vi "IQramp.vi"(8 "Q counter":fxp<+/-,14,14> format="%#_8f", 9 "I counter":fxp<+/-,13,13> format="%#_8f", 10 "cos":fxp<+/-,16,0>, 11 "sin":fxp<+/-,16,0>) -> (0 "Q counter out":fxp<+/-,14,14>, 1 "I counter out":fxp<+/-,13,13>, 3 "signal":i16)   [LabVIEW 2013]
uses:
  <vilib>/rvi/FXPMathLib/FxpConvert/subVIs/nifxpmath_Convert_SimConfig.ctl
  <vilib>/fxp/LVFixedPointQuantizationPolicyTypeDef.ctl
  <vilib>/fxp/LVFixedPointOverflowPolicyTypeDef.ctl
  <vilib>/rvi/FXPMathLib/FxpConvert/simVIs/DllFxpConvertTemp_sub.vi
  <vilib>/rvi/FXPMathLib/FxpInterpret/XNode/nifxpmath_Interpret.xnode
  <vilib>/rvi/FXPMathLib/FxpConvert/XNode/nifxpmath_Convert.xnode
  <vilib>/rvi/FXPMathLib/FxpMul/XNode/nifxpmath_Multiplier.xnode
  <vilib>/rvi/FXPMathLib/FxpSub/XNode/nifxpmath_Sub.xnode
  <vilib>/rvi/FXPMathLib/FxpAdd/XNode/nifxpmath_Add.xnode
  <vilib>/rvi/FXPMathLib/sim/FxpSim.dll
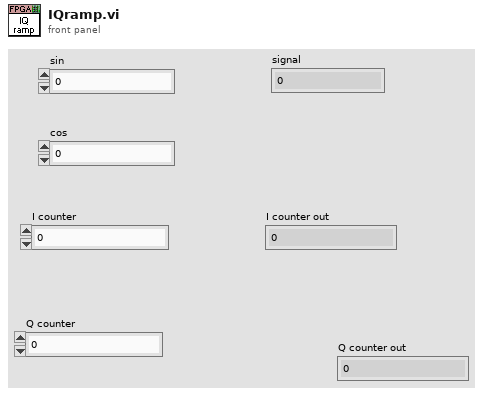
[diagram p1: front panel]
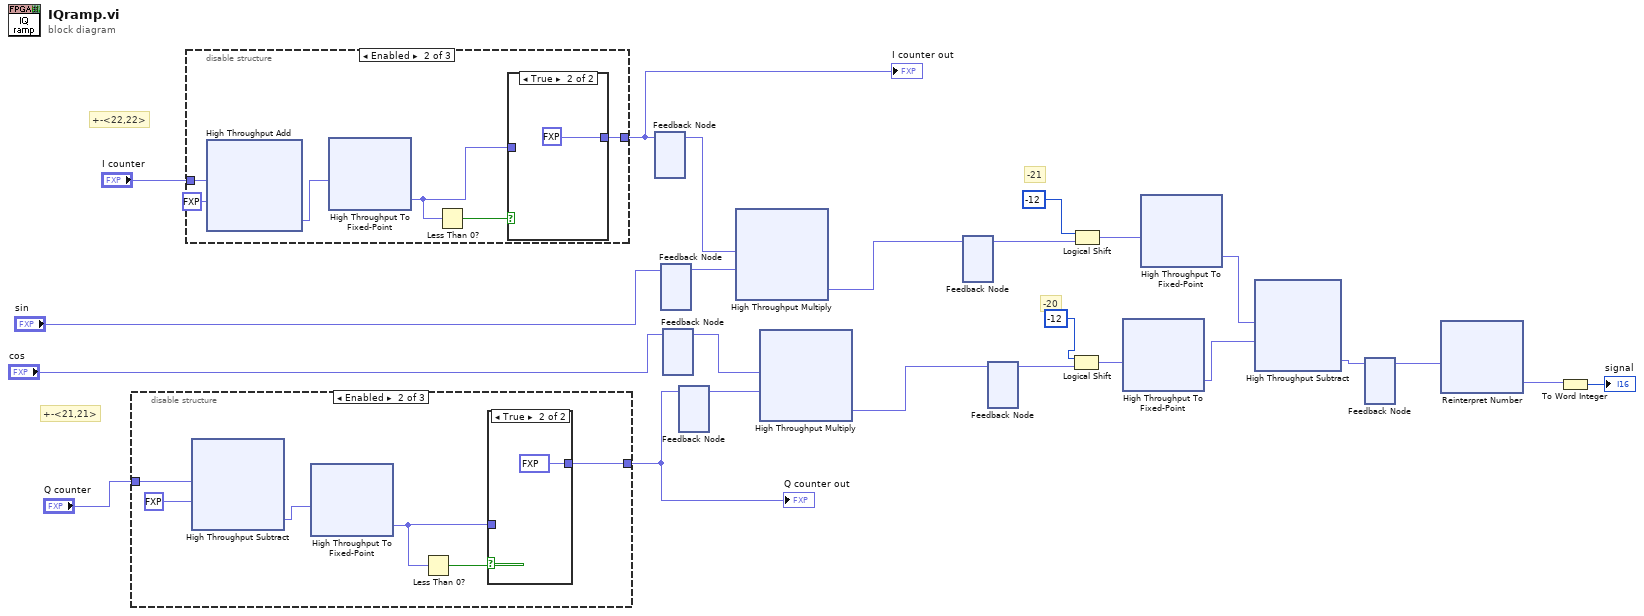
[diagram p0: block diagram]
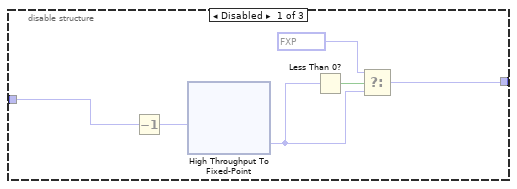
[diagram p2: hidden frame]
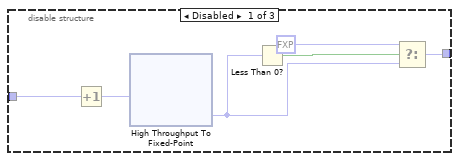
[diagram p5: hidden frame]
diagram:
  # "-20"
  # "-21"
  # "+-<21,21>"
  # "+-<22,22>"
  n1 = disable-structure shown="Enabled" {
    disable-tunnel: "Q counter" -> [w27 w55 _]
    disable-tunnel: [w25 w56 _] -> w1
    frame Disabled {
      n2 = Decrement(x=w27) -> (x-1=w28:fxp<+/-,15,15>)
      n3 = xnode "High Throughput To Fixed-Point"("x"=w28) -> ("y"=w30:fxp<+/-,21,21>)
      n4 = Less Than 0?(x=w30) -> (x < 0?=w29:bool)
      n5 = Select(t=fxp<+/-,21,21> 1048575.0 ("Q counter"), s=w29, f=w30) -> (s? t:f=w25:fxp<+/-,21,21>)
    }
    frame Enabled {
      n6 = xnode "High Throughput Subtract"("x"=w55, "y"=fxp<+/-,14,14> 1.0 ("Q counter")) -> ("x-y"=w53:fxp<+/-,14,14>)
      n7 = xnode "High Throughput To Fixed-Point"("x"=w53) -> ("y"=w57:fxp<+/-,14,14>)
      n8 = Less Than 0?(x=w57) -> (x < 0?=w58:bool)
      n9 = case shown="True" w58 {
        tunnel: w57 -> [w59 _]
        tunnel: [w59 fxp<+/-,14,14> 8191.0 ("Q counter")] -> w56
        frame False {
        }
        frame True {
        }
      }
    }
    frame Disabled {
    }
  }
  "Q counter out" <- w1
  n10 = disable-structure shown="Enabled" {
    disable-tunnel: "I counter" -> [w88 w112 _]
    disable-tunnel: [w83 w115 _] -> w2
    frame Disabled {
      n11 = Increment(x=w88) -> (x+1=w87:fxp<+/-,14,14>)
      n12 = xnode "High Throughput To Fixed-Point"("x"=w87) -> ("y"=w85:fxp<+/-,22,22>)
      n13 = Less Than 0?(x=w85) -> (x < 0?=w86:bool)
      n14 = Select(t=fxp<+/-,22,22> 0.0, s=w86, f=w85) -> (s? t:f=w83:fxp<+/-,22,22>)
    }
    frame Enabled {
      n15 = xnode "High Throughput Add"("x"=w112, "y"=fxp<+/-,13,13> 1.0 ("I counter")) -> ("x+y"=w113:fxp<+/-,13,13>)
      n16 = xnode "High Throughput To Fixed-Point"("x"=w113) -> ("y"=w116:fxp<+/-,13,13>)
      n17 = Less Than 0?(x=w116) -> (x < 0?=w114:bool)
      n18 = case shown="True" w114 {
        tunnel: w116 -> [w117 _]
        tunnel: [w117 fxp<+/-,13,13> 0.0 ("t")] -> w115
        frame False {
        }
        frame True {
        }
      }
    }
    frame Disabled {
    }
  }
  "I counter out" <- w2
  n19 = feedback #1() -> (w8:fxp<+/-,13,13>)  [unwired: 1 in]
  n20 = feedback-in #1(w2) -> ()
  n21 = feedback #2() -> (w6:fxp<+/-,16,0>)  [unwired: 1 in]
  n22 = feedback-in #2("sin") -> ()
  n23 = feedback #3() -> (w3:fxp<+/-,16,0>)  [unwired: 1 in]
  n24 = feedback-in #3("cos") -> ()
  n25 = feedback #4() -> (w5:fxp<+/-,14,14>)  [unwired: 1 in]
  n26 = feedback-in #4(w1) -> ()
  n27 = xnode "High Throughput Multiply"("x"=w8, "y"=w6) -> ("x*y"=w10:fxp<+/-,29,13>)
  n28 = xnode "High Throughput Multiply"("x"=w3, "y"=w5) -> ("x*y"=w9:fxp<+/-,30,14>)
  n29 = feedback-in #5(w10) -> ()
  n30 = feedback #5() -> (w16:fxp<+/-,29,13>)  [unwired: 1 in]
  n31 = feedback #6() -> (w15:fxp<+/-,30,14>)  [unwired: 1 in]
  n32 = feedback-in #6(w9) -> ()
  n33 = Logical Shift(y=i16 -12, x=w15) -> (x << y=w21:fxp<+/-,30,14>)
  n34 = Logical Shift(y=i16 -12, x=w16) -> (x << y=w23:fxp<+/-,29,13>)
  n35 = xnode ("High Throughput To Fixed-Point")("x"=w21) -> ("y"=w18:fxp<+/-,15,1>)
  n36 = xnode ("High Throughput To Fixed-Point")("x"=w23) -> ("y"=w20:fxp<+/-,15,1>)
  n37 = xnode "High Throughput Subtract"("x"=w20, "y"=w18) -> ("x-y"=w14:fxp<+/-,16,1>)
  n38 = feedback #7() -> (w12:fxp<+/-,16,1>)  [unwired: 1 in]
  n39 = feedback-in #7(w14) -> ()
  n40 = xnode "Reinterpret Number"("x"=w12) -> ("y"=w11:fxp<+/-,16,16>)
  n41 = To Word Integer(number=w11) -> (16bit integer=→"signal":i16)
